vi "From Variant.vi"(8 "Error In":errorcluster, 10 "Variant":variant, 11 "TD Path In":refnum<class "Path.lvclass">) -> (0 "Error Out":errorcluster, 3 "TD Path Out":refnum<class "Path.lvclass">)   [LabVIEW 2017, in "Tree API.lvlib" / "Path.lvclass"]
doc: "Dynamic dispatch interface for conversion of variant LV data to Tree Data classes."
uses:
  Path.lvclass
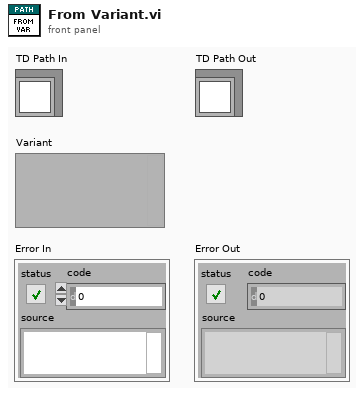
[diagram p1: front panel]
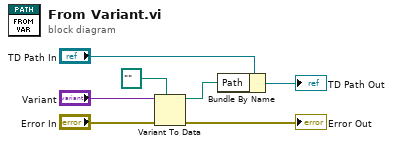
[diagram p0: block diagram]
diagram:
  n1 = Variant To Data(error in="Error In", type=path "" ("Path"), Variant="Variant") -> (data=w3:path, error out=→"Error Out":errorcluster)
  n2 = Bundle By Name(cluster="TD Path In", "Path"=w3) -> (→"TD Path Out":refnum<class "Path.lvclass">)
